vi "ficheros.vi"() -> ()   [LabVIEW 2020]
uses:
  <vilib>/ErrorRing/Error Ring.xnode
panel:
  in  "Nombre del Archivo":string
  in  "Formato":string(combo)
  in  "Direccion":path
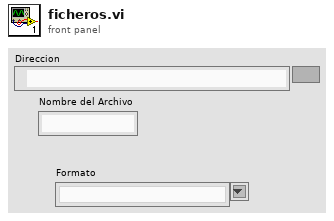
[diagram p1: front panel]
types:
  T1 = enum16{"open", "replace", "create", "open or create", "replace or create", "replace or create with confirmation"}
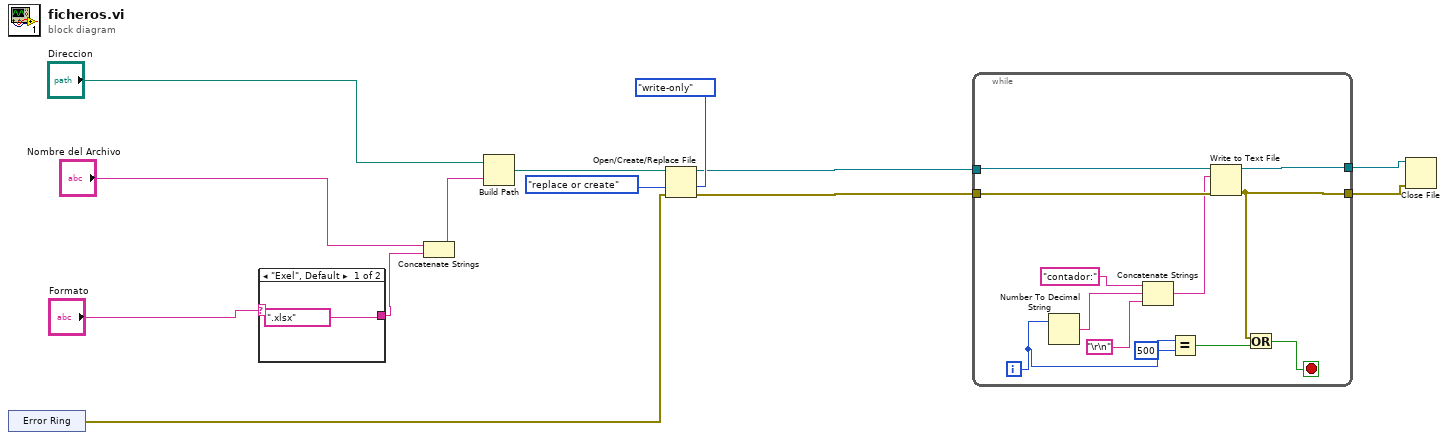
[diagram p0: block diagram]
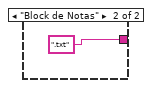
[diagram p2: hidden frame]
diagram:
  n1 = xnode "Error Ring"() -> ("error out"=w5:errorcluster)
  n2 = case shown="\"Exel\", Default" "Formato" {
    tunnel: [".xlsx" ".txt"] -> w10
    frame "Exel", Default {
    }
    frame "Block de Notas" {
    }
  }
  n3 = Concatenate Strings("Nombre del Archivo", w10) -> (w9:string)
  n4 = Build Path(base path="Direccion", name or relative path=w9) -> (appended path=w8:path)
  n5 = Open/Create/Replace File(file path (use dialog)=w8, error in=w5, operation (0:open)=T1."replace or create", access (0:read/write)=enum16{"read/write", "read-only", "write-only"}."write-only") -> (refnum out=w4:refnum<file>, error out=w3:errorcluster)  [unwired: 2 in, 1 out]
  n6 = while {
    tunnel: w4 -> [w27]
    tunnel: w3 -> [w26]
    tunnel: [w25] -> w2
    tunnel: [w21] -> w1
    i -> [w20]
    stop <- w17 stop-if-true
    n7 = Number To Decimal String(number=w20) -> (decimal integer string=w23:string)  [unwired: 1 in]
    n8 = Concatenate Strings("contador:", w23, "\r\n") -> (w16:string)
    n9 = Equal?(x=w20, y=500) -> (x = y?=w18:bool)
    n10 = Write to Text File(file (use dialog)=w27, text=w16, error in=w26) -> (refnum out=w25:refnum<file>, error out=w21:errorcluster)  [unwired: 1 in, 1 out]
    n11 = Or(x=w21, y=w18) -> (x .or. y?=w17:bool)
  }
  n12 = Close File(refnum=w2, error in=w1) -> ()  [unwired: 2 out]
